vi "Event Nested.vi"(8 "Alias":string, 10 "Msg Strategy":refnum<class "Msg Strategy.lvclass">, 11 "Base Queue jettl in":refnum<class "Base Queue jettl.lvclass">) -> (3 "Base Queue jettl out":refnum<class "Base Queue jettl.lvclass">)   [LabVIEW 2021, in "jettl.lvlib" / "Base Queue jettl.lvlib" / "Base Queue jettl.lvclass"]
uses:
  Base Queue jettl.lvclass
  Msg Strategy/Msg Strategy.lvclass
  Base Queue jettl.lvclass/Base Queue jettl.ctl
  jettl.lvlib
  Queue Mailbox/Queue Mailbox.lvlib
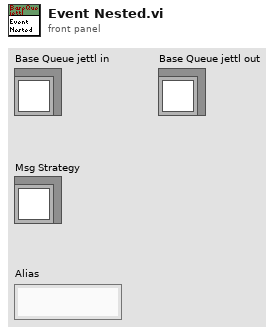
[diagram p1: front panel]
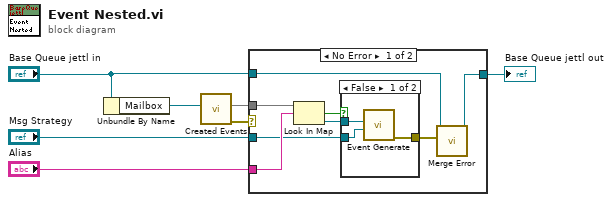
[diagram p0: block diagram]
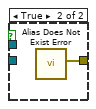
[diagram p2: hidden frame]
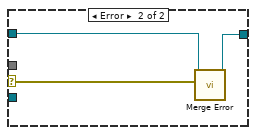
[diagram p3: hidden frame]
diagram:
  n1 = Unbundle By Name("Base Queue jettl in") -> ("Mailbox"=w6:refnum<data-value>)
  n2 = call "Created Events.vi"("Queue Mailbox"=w6) -> ("error out"=w4:errorcluster, "Event"=w5:map{string, refnum<data-value>})  [unwired: 9 in]
  n3 = case shown="No Error" w4 {
    selector: w4 -> [_ w20]
    tunnel: "Alias" -> [w12 _]
    tunnel: "Msg Strategy" -> [w11 _]
    tunnel: [w10 w21] -> w1
    tunnel: "Base Queue jettl in" -> [w9 w22]
    tunnel: w5 -> [w8 _]
    frame No Error {
      n4 = Look In Map(map=w8, key=w12) -> (key not found?=w14:bool, value=w15:refnum<data-value>)  [unwired: 1 in]
      n5 = case shown="False" w14 {
        tunnel: [w16 w19] -> w13
        tunnel: w11 -> [w17 _]
        tunnel: w15 -> [w18 _]
        frame False {
          n6 = call "Event Generate.vi"("Msg Strategy"=w17, "Event"=w18) -> ("error out"=w16:errorcluster)  [unwired: 9 in]
        }
        frame True {
          n7 = call "Alias Does Not Exist Error.vi"() -> ("Error"=w19:errorcluster)  [unwired: 11 in]
        }
      }
      n8 = call-dynamic "Merge Error.vi"("Error"=w13, "Base Queue jettl in"=w9) -> ("Base Queue jettl out"=w10:refnum<class "Base Queue jettl.lvclass">)  [unwired: 9 in]
    }
    frame Error {
      n9 = call-dynamic "Merge Error.vi"("Error"=w20, "Base Queue jettl in"=w22) -> ("Base Queue jettl out"=w21:refnum<class "Base Queue jettl.lvclass">)  [unwired: 9 in]
    }
  }
  "Base Queue jettl out" <- w1
